vi "FM_RTL-SDR_RX_atan2_COM.vi"() -> (3 "Calculation Time (s)":dbl)   [LabVIEW 2013]
doc: "Demonstrates how to use the MATLAB script node. The m-file script is used to calculate the data and the resulting fractal is displayed on the front panel. The MathWorks, Inc. MATLAB (R) Application Software version 5.0 or later must be installed and properly licensed in order to run this VI."
uses:
  <vilib>/Waveform/WDTFileIO.llb/Read Waveform from File.vi
panel:
  in  "FMDemodRTLSDR_COM.IClass1":refnum<k7>
  out "data":dbl[][](array[numeric])
  in  "file path":path=path "D:/File/Recoder_Data_IQIQ"
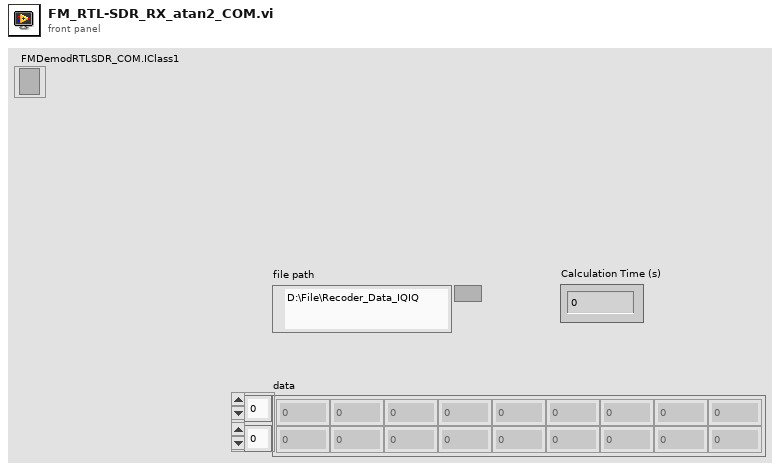
[diagram p1: front panel]
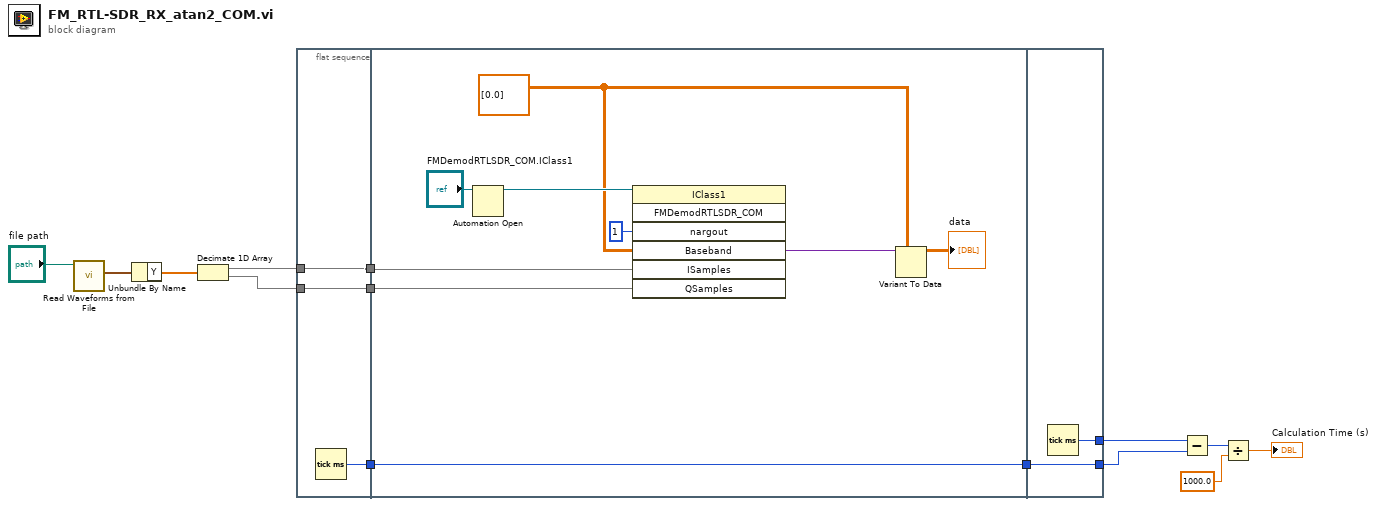
[diagram p0: block diagram]
diagram:
  n1 = call-poly <vilib>:"Read Waveforms from File.vi"("file path (dialog if empty)"="file path") -> ("first waveform in record"=w7:waveform(dbl))  [unwired: 5 in, 3 out]
  n2 = Unbundle By Name(w7) -> ("Y"=w5:dbl[])
  n3 = Decimate 1D Array(w5) -> (w4:dbl[], w2:dbl[])
  n4 = flat-sequence {
    tunnel: [w17] -> w8
    tunnel: w4 -> [w16]
    tunnel: [w16] -> w3
    tunnel: w2 -> [w15]
    tunnel: [w15] -> w1
    tunnel: [w26] -> w14
    tunnel: w8 -> [w26]
    tunnel: w3 -> [w23]
    tunnel: w1 -> [w22]
    tunnel: w14 -> [w27]
    tunnel: [w28] -> w11
    tunnel: [w27] -> w10
    frame #0 {
      n5 = Tick Count (ms)() -> (millisecond timer value=w17:u32)
    }
    frame #1 {
      w21 = dbl[][] [[0.0]]
      n6 = Automation Open(Automation Refnum="FMDemodRTLSDR_COM.IClass1") -> (Automation Refnum=w24:refnum<k7>)  [unwired: 3 in, 1 out]
      n7 = invoke class="IClass1" method="FMDemodRTLSDR_COM"(reference=w24, "nargout"=1, "Baseband"=w21, "ISamples"=w23, "QSamples"=w22) -> ("Baseband"=w19:variant)  [unwired: 2 in, 6 out]
      n8 = Variant To Data(type=w21, Variant=w19) -> (data=→"data":dbl[][])  [unwired: 1 in, 1 out]
    }
    frame #2 {
      n9 = Tick Count (ms)() -> (millisecond timer value=w28:u32)
    }
  }
  n10 = Subtract(x=w11, y=w10) -> (x-y=w12:u32)
  n11 = Divide(x=w12, y=1000.0) -> (x/y=→"Calculation Time (s)":dbl)
